vi "JAS-Color Sensor V3 Get Color.vi"(8 "error in (no error)":errorcluster, 11 "ColorSensorDevRef":T1={"I2CDevRef"={"DevStatus"={"status"=FALSE, "code"=0, "source"=""}, "Device Address"=0, "Handle"=0, "I2C Bus"=enum."Invalid"}} {"I2CDevRef"."Device Address" format="%.0x"}) -> (0 "error out":errorcluster, 1 "Normalized Color":cluster{"R":dbl, "G":dbl, "B":dbl}, 2 "Color":u32(colorbox), 3 "ColorSensorDevRef out":T1={"I2CDevRef"={"DevStatus"={"status"=FALSE, "code"=0, "source"=""}, "Device Address"=0, "Handle"=0, "I2C Bus"=enum."Invalid"}} {"I2CDevRef"."Device Address" format="%.0x"})   [LabVIEW 2019]
uses:
  <vilib>/Rock Robotics/WPI/ThirdParty/REV Robotics/Color SensorV3/Typedef/Color Sensor V3 DevRef.ctl
  <vilib>/Rock Robotics/WPI/I2C/WPI_I2CDevRef.ctl
  <vilib>/Rock Robotics/SystemInterfaces/i2clib/i2c_bus.ctl
panel:
  in  "RedGain":dbl format="%10.4f"
  in  "GreenGain":dbl format="%10.4f"
  in  "BlueGain":dbl format="%10.4f"
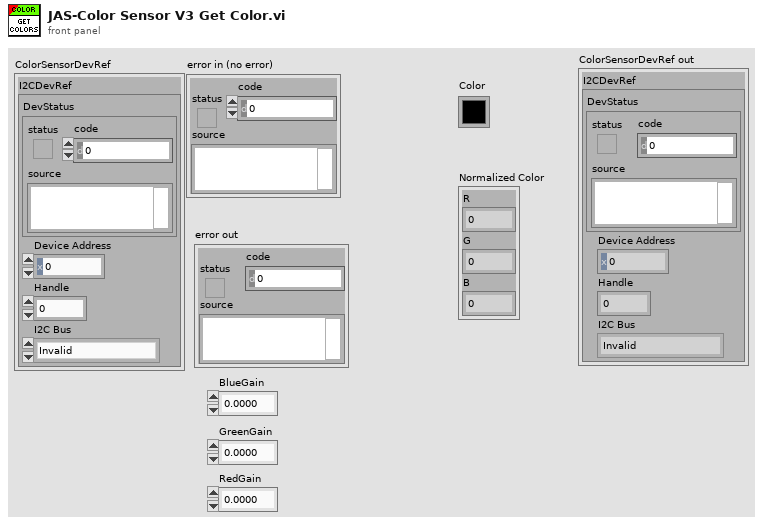
[diagram p1: front panel]
types:
  T1 = typedef "Color Sensor V3 DevRef.ctl" = cluster{"I2CDevRef":T2}
  T2 = typedef "WPI_I2CDevRef.ctl" = cluster{"DevStatus":errorcluster, "Device Address":u8, "Handle":i32, "I2C Bus":T3}
  T3 = typedef "i2c_bus.ctl" = enum16{"I2C On-Board", "I2C MXP", "Invalid"}
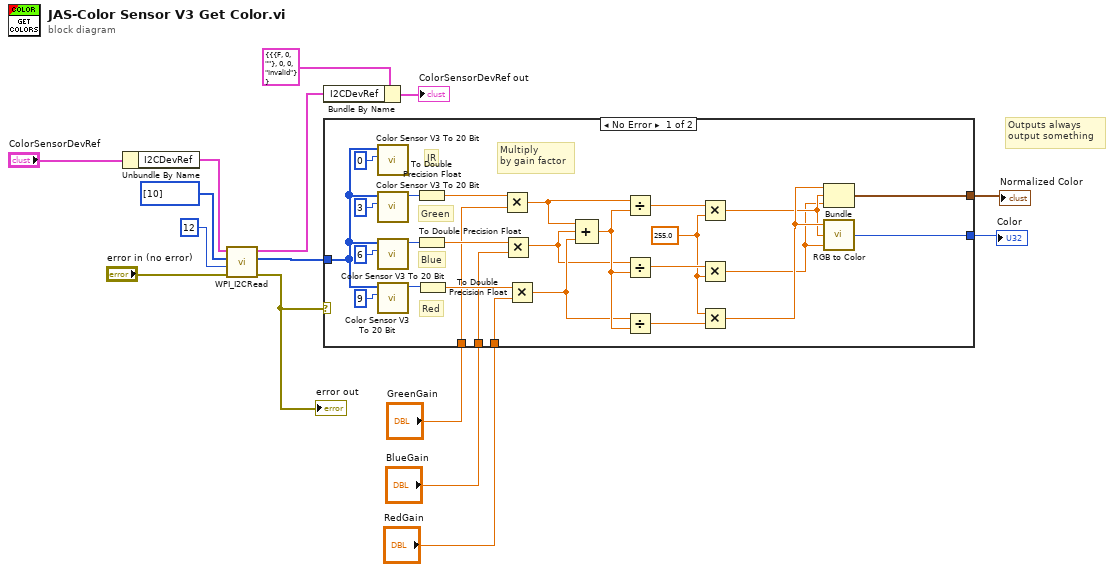
[diagram p0: block diagram]
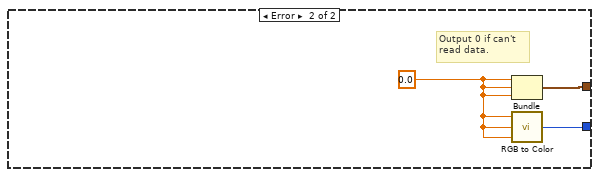
[diagram p2: hidden frame]
diagram:
  # "Outputs always\noutput something"
  n1 = Unbundle By Name("ColorSensorDevRef") -> ("I2CDevRef"=w12:T2)
  n2 = call <vilib>:"WPI_I2CRead.vi"("error in (no error)"="error in (no error)", "I2CBytesToRead"=u8 12, "I2CRegister"=u8[] [10], "I2CDevRef"=w12) -> ("error out"=w10:errorcluster, "Data Out"=w9:u8[], "I2CDevRef"=w7:T2)  [unwired: 5 in]
  "error out" <- w10
  n3 = Bundle By Name(cluster=T1 {"I2CDevRef"={"DevStatus"={"status"=FALSE, "code"=0, "source"=""}, "Device Address"=0, "Handle"=0, "I2C Bus"=enum."Invalid"}} ("ColorSensorDevRef 2"), "I2CDevRef"=w7) -> (→"ColorSensorDevRef out":T1)
  n4 = case shown="No Error" w10 {
    tunnel: w9 -> [w42 _]
    tunnel: "GreenGain" -> [w20 _]
    tunnel: "BlueGain" -> [w19 _]
    tunnel: "RedGain" -> [w18 _]
    tunnel: [w17 w45] -> w2
    tunnel: [w16 w44] -> w1
    frame No Error {
      w33 = 255.0 ("y")
      # "Multiply\nby gain factor"
      # "Red"
      # "Blue"
      # "Green"
      # "IR"
      n5 = call <vilib>:"Color Sensor V3 To 20 Bit.vi"("index (0)"=0 ("index"), "array"=w42) -> ()  [unwired: 9 in, 1 out]
      n6 = call <vilib>:"Color Sensor V3 To 20 Bit.vi"("index (0)"=3 ("index"), "array"=w42) -> ("Result"=w29:u32)  [unwired: 9 in]
      n7 = call <vilib>:"Color Sensor V3 To 20 Bit.vi"("index (0)"=6 ("index"), "array"=w42) -> ("Result"=w28:u32)  [unwired: 9 in]
      n8 = call <vilib>:"Color Sensor V3 To 20 Bit.vi"("index (0)"=9 ("index"), "array"=w42) -> ("Result"=w27:u32)  [unwired: 9 in]
      n9 = To Double Precision Float(number=w29) -> (double precision float=w25:dbl)
      n10 = To Double Precision Float(number=w28) -> (double precision float=w22:dbl)
      n11 = To Double Precision Float(number=w27) -> (double precision float=w24:dbl)
      n12 = Multiply(x=w25, y=w20) -> (x*y=w26:dbl)
      n13 = Multiply(x=w22, y=w19) -> (x*y=w21:dbl)
      n14 = Multiply(x=w24, y=w18) -> (x*y=w23:dbl)
      n15 = Compound Arithmetic op=ADD(w26, w21, w23) -> (w37:dbl)
      n16 = Divide(x=w26, y=w37) -> (x/y=w36:dbl)
      n17 = Divide(x=w21, y=w37) -> (x/y=w35:dbl)
      n18 = Divide(x=w23, y=w37) -> (x/y=w34:dbl)
      n19 = Multiply(x=w36, y=w33) -> (x*y=w31:dbl)
      n20 = Multiply(x=w35, y=w33) -> (x*y=w30:dbl)
      n21 = Multiply(x=w33, y=w34) -> (x*y=w32:dbl)
      n22 = Bundle(w32, w31, w30) -> (w17:cluster{dbl, dbl, dbl})  [unwired: 1 in]
      n23 = call <vilib>:"RGB to Color.vi"("B"=w30, "G"=w31, "R"=w32) -> ("Color"=w16:u32)
    }
    frame Error {
      w43 = 0.0 ("y")
      # "Output 0 if can't \nread data."
      n24 = Bundle("y"=w43, "y"=w43, "y"=w43) -> (w45:cluster{"y":dbl, "y":dbl, "y":dbl})  [unwired: 1 in]
      n25 = call <vilib>:"RGB to Color.vi"("B"=w43, "G"=w43, "R"=w43) -> ("Color"=w44:u32)
    }
  }
  "Color" <- w1
  "Normalized Color" <- w2
